vi "unmarshalling.vi"(7 "Type":variant, 8 "error in (no error)":errorcluster, 10 "String":string, 11 "Serializer in":refnum<class "Serializer.erdosmiller-TOML.lvclass">) -> (0 "error out":errorcluster, 2 "Variant":variant, 3 "Serializer":refnum<class "Serializer.erdosmiller-TOML.lvclass">)   [LabVIEW 2019, in "OpenSerializer.erdosmiller-TOML.lvlib" / "Serializer.erdosmiller-TOML.lvclass"]
uses:
  Serializer.erdosmiller-TOML.lvclass
  <vilib>/Erdos Miller/LV-TOML/LV-TOML.lvlib
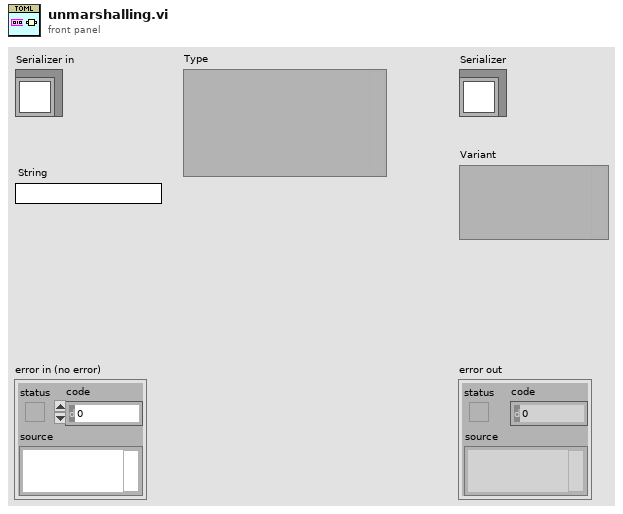
[diagram p1: front panel]
types:
  T1 = typedef "LV-TOML.lvlib/TOML Value.ctl" = cluster{"\\type":enum16{"Table", "Array", "String", "Integer", "Float", "Boolean", "Offset Date-Time", "Local Date-Time", "Local Date", "Local Time"}, "ÿýÿýÿýÿýÿýÿþÿýÿýÿý%LV-TOML.lvlib:TOML Key-Value Pair.ctlÿýÿýÿýÿýÿýÿþÿýÿýÿýLV-TOML.lvlib:TOML Value.ctl$":variant}
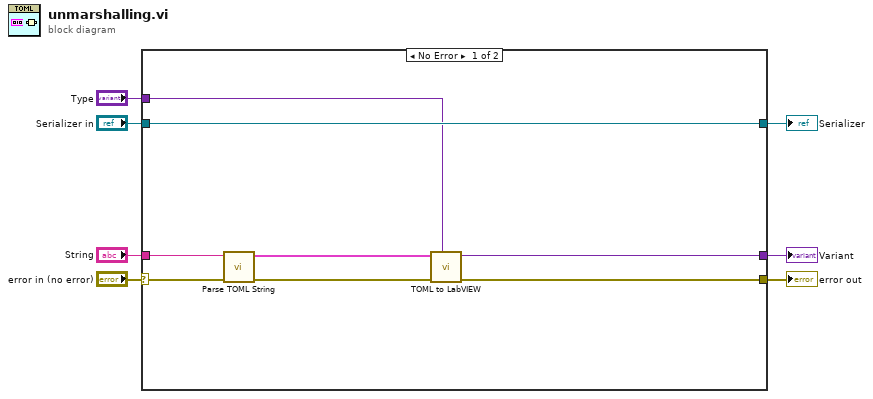
[diagram p0: block diagram]
diagram:
  n1 = case shown="No Error" "error in (no error)" {
    selector: "error in (no error)" -> [w14 w16]
    tunnel: "Serializer in" -> [w15 w17]
    tunnel: "String" -> [w13 _]
    tunnel: [w15 w17] -> w5
    tunnel: [w10 w16] -> w4
    tunnel: [w9 _] -> w3
    tunnel: "Type" -> [w8 _]
    frame No Error {
      n2 = call <vilib>:"Parse TOML String.vi"("error in (no error)"=w14, "String"=w13) -> ("error out"=w11:errorcluster, "Value"=w12:T1)  [unwired: 8 in]
      n3 = call <vilib>:"TOML to LabVIEW.vi"("Default Value"=w8, "error in (no error)"=w11, "TOML Value"=w12) -> ("error out"=w10:errorcluster, "LV Value"=w9:variant)  [unwired: 7 in]
    }
    frame Error {
    }
  }
  "error out" <- w4
  "Serializer" <- w5
  "Variant" <- w3
